vi "eodrecorder.vi"() -> ()   [LabVIEW 2014]
uses:
  eodrecorderstates.ctl
  Control 1.ctl
  <vilib>/Utility/error.llb/DialogType.ctl
  <vilib>/_DAQmxBase/Internals/DAQmxBase Create Channel (AI-Voltage-Basic).vi
  <vilib>/_DAQmxBase/Internals/DAQmxBase Timing (Sample Clock).vi
  <vilib>/_DAQmxBase/Internals/DAQmxBase Read (Analog 2D DBL NChan NSamp).vi
panel:
  out "String 2":string
  out "String":string
  out "Tab Control":enum32{"Live Data", "Edit Data", "View Data"}(tab)
  out "WaveformData":T1
  out "# Pretrigger Samples\nAcquired":i32
  out "Pre-Trigger Error Indicator":bool caption="Error Indicator\n(Indicates if trigger occurs before\npre-trigger samples were acquired)"
  in  "Channel Index":i32
  in  "Pretrigger Samples":i32
  in  "Threshold":sgl
  out "Waveform Graph":dbl[][](graph) caption="Measurement"
  in  "SampleRate":dbl=10000.0
  in  "LiveDataMode":bool
  in  "NumSamptoGrab":i32
  in  "Capture":bool
  in  "Stop":bool
  in  "Open Data":bool
  # "Off"
  # "On"
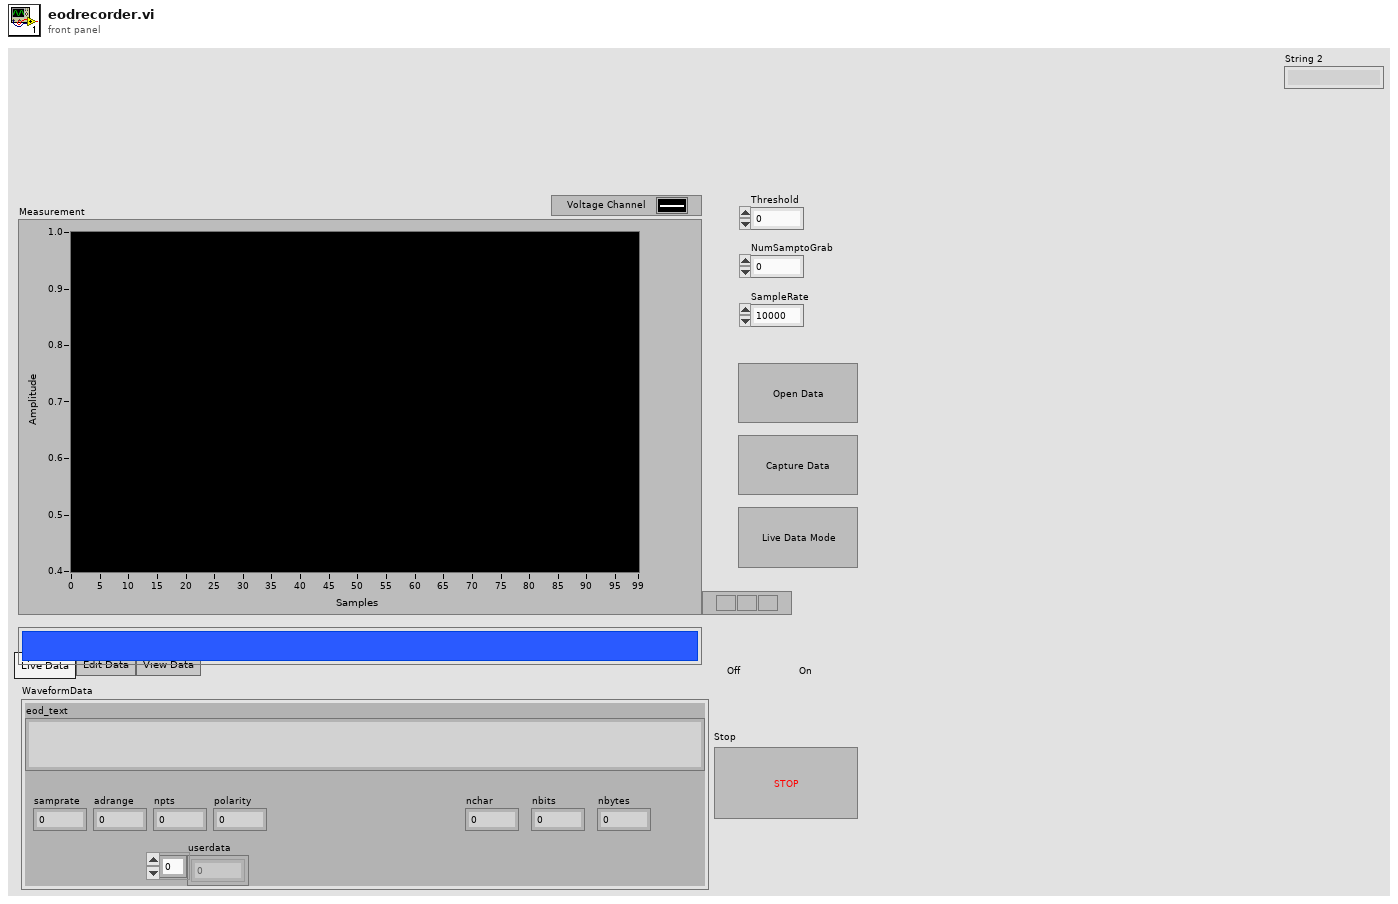
[diagram p1: front panel]
types:
  T1 = cluster{"eod_text":string, "nchar":i32, "nbits":i32, "nbytes":i32, "polarity":i32, "samprate":i32, "adrange":dbl, "userdata":dbl[], "npts":i32, "Wave":dbl[]}
  T2 = cluster{"data":dbl[][], "task ":refnum<k21>, "error ":errorcluster, "Channel":tag, "Min":dbl, "Max":dbl, "Srate":dbl, "WaveformData":cluster{"eod_text":string, "nchar":i32, "nbits":i32, "nbytes":i32, "polarity":i32, "samprate":i32, "adrange":dbl, "userdata":dbl[], "npts":i32, "Wave":dbl[]}}
  T3 = typedef "eodrecorderstates.ctl" = enum16{"stop", "initialize", "live data", "capture data", "analyze data", "open data", "display opened data", "write to file"}
  T4 = typedef "Control 1.ctl" = enum32{"Live Data", "Edit Data", "View Data"}
  T5 = enum16{"Rising Edge", "Falling Edge", "Above Level", "Below Level", "When Inside Window", "When Outside Window"}
  T6 = enum16{"open", "replace", "create", "open or create", "replace or create", "replace or create with confirmation"}
  T7 = typedef "DialogType.ctl" = u16
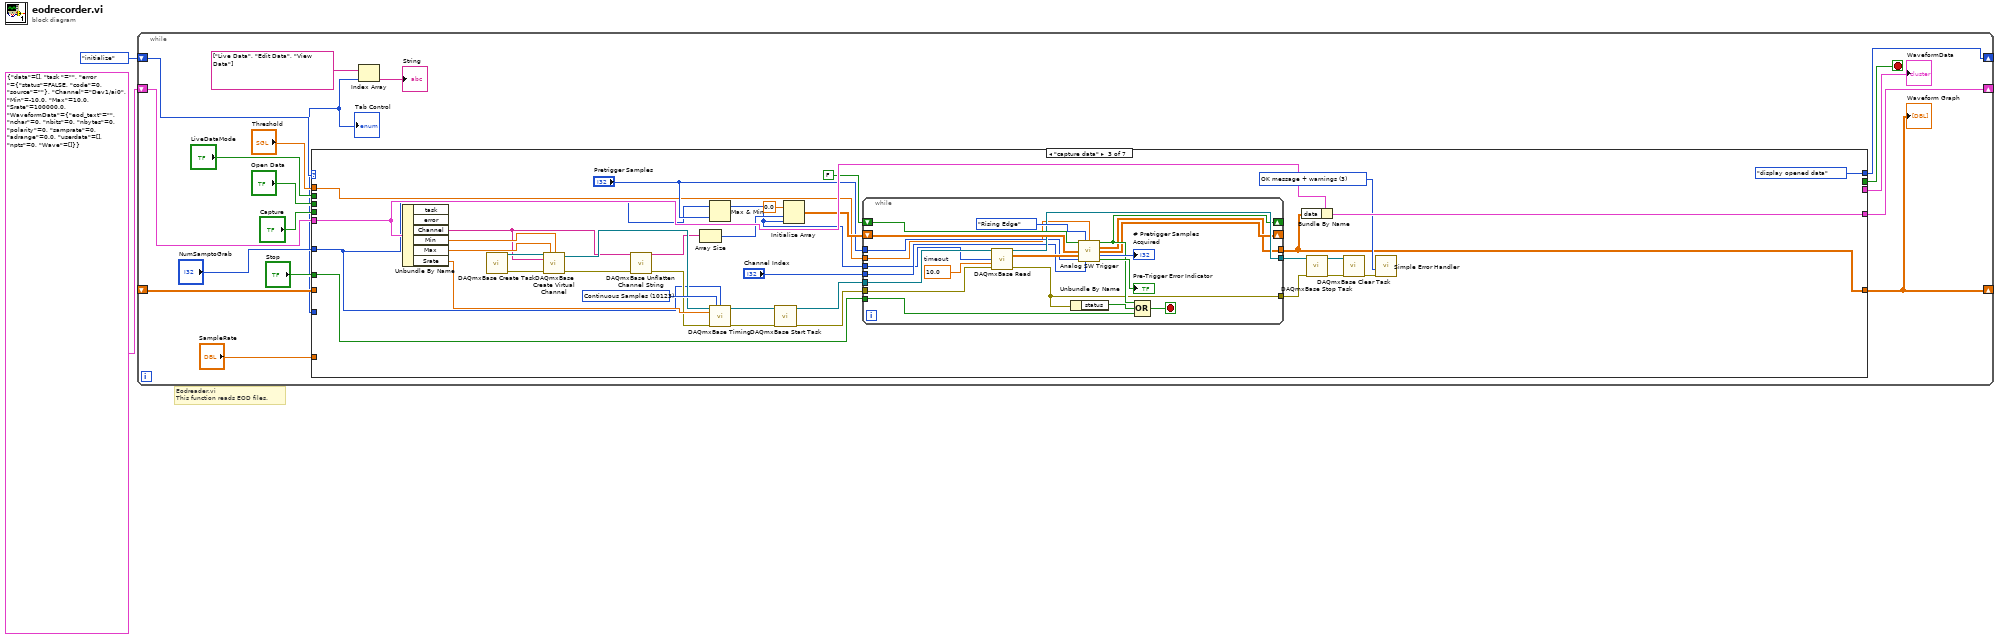
[diagram p0: block diagram]
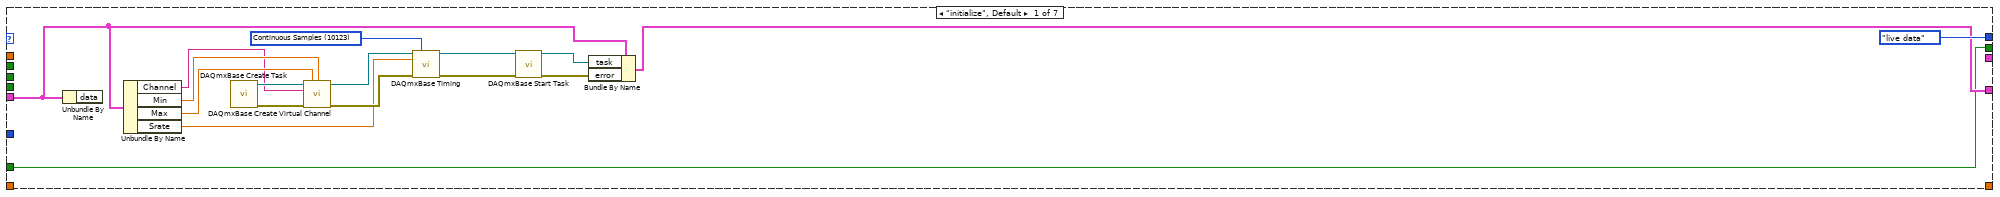
[diagram p2: hidden frame]
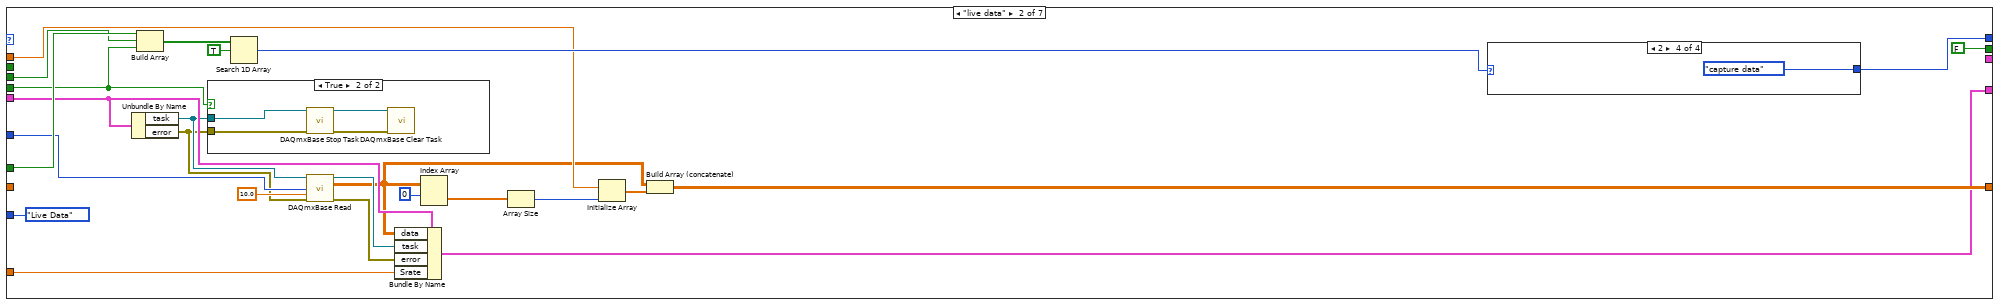
[diagram p3: hidden frame]
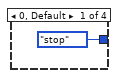
[diagram p5: hidden frame]
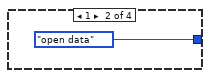
[diagram p6: hidden frame]
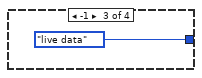
[diagram p7: hidden frame]
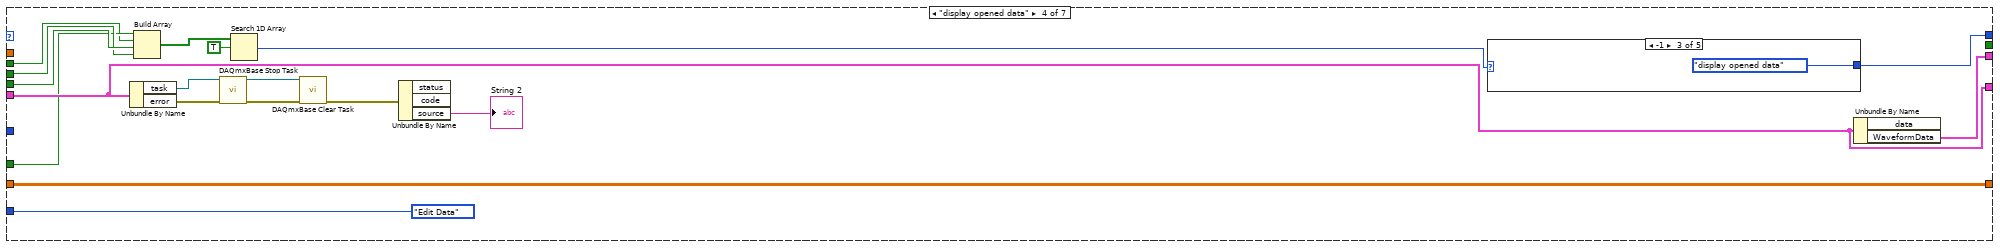
[diagram p8: hidden frame]
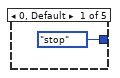
[diagram p9: hidden frame]
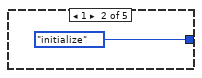
[diagram p10: hidden frame]
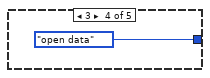
[diagram p11: hidden frame]
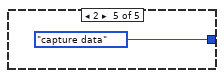
[diagram p12: hidden frame]
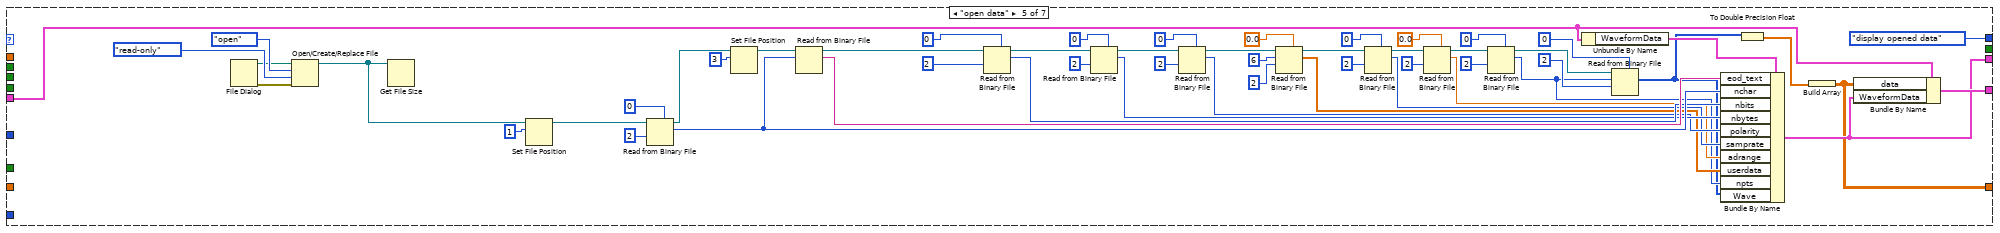
[diagram p13: hidden frame]
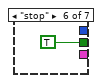
[diagram p14: hidden frame]
diagram:
  # "Eodreader.vi\nThis function reads EOD files."
  n1 = while {
    shift-right: [w19] -> _
    shift-left: eodrecorderstates."initialize" ("Enum") -> [w8]
    shift-right: [w17] -> _
    shift-left: T2 {"data"=[], "task "="", "error "={"status"=FALSE, "code"=0, "source"=""}, "Channel"="Dev1/ai0", "Min"=-10.0, "Max"=10.0, "Srate"=100000.0, "WaveformData"={"eod_text"="", "nchar"=0, "nbits"=0, "nbytes"=0, "polarity"=0, "samprate"=0, "adrange"=0.0, "userdata"=[], "npts"=0, "Wave"=[]}} -> [w14]
    shift-right: [w7] -> _
    shift-left: _ -> [w6]
    stop <- w20 stop-if-true
    n2 = case shown="\"capture data\"" w8 {
      tunnel: [w34 FALSE _ _ _ TRUE _] -> w20
      tunnel: [eodrecorderstates."live data" ("Enum") w61 eodrecorderstates."display opened data" ("Enum") w142 eodrecorderstates."display opened data" ("Enum") _ _] -> w19
      tunnel: "Stop" -> [w34 w60 w74 w136 _ _ _]
      tunnel: w14 -> [w35 w56 w103 w143 w151 _ _]
      tunnel: [w36 w39 w102 w143 w155 _ _] -> w17
      tunnel: [_ _ _ w144 w152 _ _] -> w16
      tunnel: "NumSamptoGrab" -> [_ w52 w71 _ _ _ _]
      tunnel: "SampleRate" -> [_ w50 _ _ _ _ _]
      tunnel: "Open Data" -> [_ w51 _ w138 _ _ _]
      tunnel: "Capture" -> [_ w47 _ w139 _ _ _]
      tunnel: "LiveDataMode" -> [_ _ _ w135 _ _ _]
      tunnel: [_ w48 w72 w128 w150 _ _] -> w7
      tunnel: "Threshold" -> [_ w49 w73 _ _ _ _]
      tunnel: w6 -> [_ _ _ w128 _ _ _]
      tunnel: [_ Control_1."Live Data" ("Tab Control") _ Control_1."Edit Data" ("Tab Control") _ _ _] -> w3
      frame "initialize", Default {
        w29 = 10123 items=["Finite Samples"=10178, "Continuous Samples"=10123] ("sample mode")
        n3 = Unbundle By Name(w35) -> ()  [unwired: 1 out]
        n4 = Unbundle By Name(w35) -> ("Channel"=w21:tag, "Min"=w26:dbl, "Max"=w25:dbl, "Srate"=w24:dbl)
        n5 = call <vilib>:"DAQmxBase Create Task.vi"() -> ("task out"=w32:refnum<k21>, "error out"=w33:errorcluster)  [unwired: 5 in, 9 out]
        n6 = call-poly <vilib>:"DAQmxBase Create Virtual Channel.vi"("task in"=w32, "maximum value"=w25, "minimum value"=w26, "physical channels"=w21, "error in"=w33) -> ("task out"=w30:refnum<k21>, "error out"=w31:errorcluster)  [unwired: 4 in, 5 out]
        n7 = call-poly <vilib>:"DAQmxBase Timing.vi"("task/channels in"=w30, "sample mode"=w29, "rate"=w24, "error in"=w31) -> ("task out"=w23:refnum<k21>, "error out"=w22:errorcluster)  [unwired: 3 in, 7 out]
        n8 = call <vilib>:"DAQmxBase Start Task.vi"("task/channels in"=w23, "error in"=w22) -> ("task out"=w28:refnum<k21>, "error out"=w27:errorcluster)  [unwired: 12 out]
        n9 = Bundle By Name(cluster=w35, "task"=w28, "error"=w27) -> (w36:T2)
      }
      frame "live data" {
        n10 = Unbundle By Name(w56) -> ("task"=w46:refnum<k21>, "error"=w45:errorcluster)
        n11 = Build Array(w60, w51, w47) -> (w59:bool[])
        n12 = case shown="True" w47 {
          tunnel: w46 -> [_ w66]
          tunnel: w45 -> [_ w65]
          frame False {
          }
          frame True {
            n13 = call <vilib>:"DAQmxBase Stop Task.vi"("task/channels in"=w66, "error in"=w65) -> ("task out"=w64:refnum<k21>, "error out"=w63:errorcluster)  [unwired: 12 in]
            n14 = call <vilib>:"DAQmxBase Clear Task.vi"("task in"=w64, "error in"=w63) -> ()  [unwired: 13 in, 1 out]
          }
        }
        n15 = Search 1D Array(1D array=w59, element=TRUE) -> (index of element=w57:i32)  [unwired: 1 in]
        n16 = call-poly <vilib>:"DAQmxBase Read.vi"("task/channels in"=w46, "number of samples per channel"=w52, "timeout"=10.0, "error in"=w45) -> ("task out"=w55:refnum<k21>, "data"=w40:dbl[][], "error out"=w54:errorcluster)  [unwired: 9 out]
        n17 = Bundle By Name(cluster=w56, "data"=w40, "task"=w55, "error"=w54, "Srate"=w50) -> (w39:T2)
        n18 = Index Array(array=w40, index (row)=0) -> (element=w42:dbl[])  [unwired: 1 in]
        n19 = Array Size(array=w42) -> (size(s)=w43:i32)
        n20 = Initialize Array(w49, w43) -> (w41:sgl[])
        n21 = Build Array (concatenate)(w40, w41) -> (w48:dbl[][])
        n22 = case shown="2" w57 {
          tunnel: [eodrecorderstates."stop" ("Enum") eodrecorderstates."open data" ("Enum") eodrecorderstates."live data" ("Enum") eodrecorderstates."capture data" ("Enum")] -> w61
          frame 0, Default {
          }
          frame 1 {
          }
          frame -1 {
          }
          frame 2 {
          }
        }
      }
      frame "capture data" {
        w79 = T7 3 items=["no dialog", "OK message", "continue or stop message", "OK message + warnings", "continue/stop + warnings"] ("type of dialog (OK msg:1)")
        w104 = 10123 items=["Finite Samples"=10178, "Continuous Samples"=10123] ("sample mode")
        n23 = Unbundle By Name(w103) -> ("Channel"=w93:tag, "Min"=w99:dbl, "Max"=w98:dbl, "Srate"=w97:dbl)  [unwired: 2 out]
        n24 = call <vilib>:"DAQmxBase Create Task.vi"() -> ("task out"=w101:refnum<k21>, "error out"=w100:errorcluster)  [unwired: 14 in]
        n25 = call-poly <vilib>:"DAQmxBase Create Virtual Channel.vi"("task in"=w101, "maximum value"=w98, "minimum value"=w99, "physical channels"=w93, "error in"=w100) -> ("task out"=w96:refnum<k21>, "error out"=w92:errorcluster)  [unwired: 9 in]
        n26 = call "DAQmxBase Unflatten Channel String.vi"("names in"=w93, "error in"=w92) -> ("names out"=w90:string[], "error out"=w91:errorcluster)  [unwired: 12 in]
        n27 = Array Size(array=w90) -> (size(s)=w89:i32)
        n28 = Max & Min(x=w71, y="Pretrigger Samples") -> (max(x,y)=w81:i32)  [unwired: 1 out]
        n29 = call-poly <vilib>:"DAQmxBase Timing.vi"("task/channels in"=w96, "sample mode"=w104, "samples per channel"=w71, "rate"=w97, "error in"=w91) -> ("task out"=w95:refnum<k21>, "error out"=w94:errorcluster)  [unwired: 2 in, 7 out]
        n30 = call <vilib>:"DAQmxBase Start Task.vi"("task/channels in"=w95, "error in"=w94) -> ("task out"=w86:refnum<k21>, "error out"=w87:errorcluster)  [unwired: 12 out]
        n31 = Initialize Array(0.0, w89, w81) -> (w85:dbl[][])
        n32 = while {
          tunnel: [w117] -> w76
          shift-right: [w116] -> _
          shift-left: FALSE ("Trigger Out") -> [w125]
          shift-right: [w110] -> _
          shift-left: w85 -> [w119]
          tunnel: w87 -> [w115]
          tunnel: w86 -> [w114]
          tunnel: "Pretrigger Samples" -> [w113]
          tunnel: "Channel Index" -> [w112]
          tunnel: w81 -> [w111]
          tunnel: [w109] -> w72
          tunnel: [w108] -> w75
          tunnel: w74 -> [w107]
          tunnel: w73 -> [w106]
          stop <- w123 stop-if-true
          w126 = 10.0  # timeout
          n33 = call-poly <vilib>:"DAQmxBase Read.vi"("task/channels in"=w114, "number of samples per channel"=w111, "timeout"=w126, "error in"=w115) -> ("task out"=w117:refnum<k21>, "data"=w120:dbl[][], "error out"=w108:errorcluster)  [unwired: 9 in]
          n34 = Unbundle By Name(w108) -> ("status"=w124:bool)
          n35 = call "Analog SW Trigger.vi"("Triggered?"=w125, "Condition"=T5."Rising Edge", "Level"=w106, "Initialized Data Array"=w119, "Input Raw Data"=w120, "Pretrigger Samples"=w113, "Index of Condition Channel"=w112) -> ("Trigger Out"=w116:bool, "Output Data (Scaled)"=w109:dbl[][], "Raw Data Out"=w110:dbl[][], "# Pretrigger Samples"=→"# Pretrigger Samples\nAcquired":i32, "Pre-Trigger Error"=→"Pre-Trigger Error Indicator":bool)  [unwired: 4 in]
          n36 = Compound Arithmetic op=OR(w116, w124, w107) -> (w123:bool)
        }
        n37 = Bundle By Name(cluster=w103, "data"=w72) -> (w102:T2)
        n38 = call <vilib>:"DAQmxBase Stop Task.vi"("task/channels in"=w76, "error in"=w75) -> ("task out"=w78:refnum<k21>, "error out"=w77:errorcluster)  [unwired: 12 in]
        n39 = call <vilib>:"DAQmxBase Clear Task.vi"("task in"=w78, "error in"=w77) -> ("error out"=w80:errorcluster)  [unwired: 13 in]
        n40 = call <vilib>:"Simple Error Handler.vi"("type of dialog (OK msg:1)"=w79, "error in (no error)"=w80) -> ()  [unwired: 3 in, 5 out]
      }
      frame "display opened data" {
        n41 = Unbundle By Name(w143) -> ("task"=w130:refnum<k21>, "error"=w129:errorcluster)
        n42 = Build Array(w136, w135, w139, w138) -> (w141:bool[])
        n43 = call <vilib>:"DAQmxBase Stop Task.vi"("task/channels in"=w130, "error in"=w129) -> ("task out"=w131:refnum<k21>, "error out"=w132:errorcluster)  [unwired: 12 in]
        n44 = Search 1D Array(1D array=w141, element=TRUE) -> (index of element=w137:i32)  [unwired: 1 in]
        n45 = call <vilib>:"DAQmxBase Clear Task.vi"("task in"=w131, "error in"=w132) -> ("error out"=w133:errorcluster)  [unwired: 13 in]
        n46 = Unbundle By Name(w133) -> ("source"=→"String 2":string)  [unwired: 2 out]
        n47 = case shown="-1" w137 {
          tunnel: [eodrecorderstates."stop" ("Enum") eodrecorderstates."initialize" ("Enum") eodrecorderstates."display opened data" ("Enum") eodrecorderstates."open data" ("Enum") eodrecorderstates."capture data" ("Enum")] -> w142
          frame 0, Default {
          }
          frame 1 {
          }
          frame -1 {
          }
          frame 3 {
          }
          frame 2 {
          }
        }
        n48 = Unbundle By Name(w143) -> ("WaveformData"=w144:T1)  [unwired: 1 out]
      }
      frame "open data" {
        n49 = File Dialog() -> (0:w199:errorcluster, 3:w200:path)  [unwired: 7 in, 2 out]
        n50 = Open/Create/Replace File(file path (use dialog)=w200, error in=w199, operation (0:open)=T6."open", access (0:read/write)=enum16{"read/write", "read-only", "write-only"}."read-only") -> (refnum out=w198:refnum<file>)  [unwired: 2 in, 2 out]
        n51 = Get File Size(file=w198) -> ()  [unwired: 1 in, 3 out]
        n52 = Set File Position(offset (in bytes) (0)=1, refnum=w198) -> (refnum out=w196:refnum<file>)  [unwired: 2 in, 1 out]
        n53 = Read from Binary File(5:u8 0, 9:2, 11:w196) -> (2:w165:u8, 3:w194:refnum<file>)  [unwired: 3 in, 2 out]
        n54 = Set File Position(offset (in bytes) (0)=3, refnum=w194) -> (refnum out=w192:refnum<file>)  [unwired: 2 in, 1 out]
        n55 = Read from Binary File(10:w165, 11:w192) -> (2:w164:string, 3:w191:refnum<file>)  [unwired: 4 in, 2 out]
        n56 = Read from Binary File(5:i8 0, 9:2, 11:w191) -> (2:w163:i8, 3:w167:refnum<file>)  [unwired: 3 in, 2 out]
        n57 = Read from Binary File(5:i8 0, 9:2, 11:w167) -> (2:w162:i8, 3:w168:refnum<file>)  [unwired: 3 in, 2 out]
        n58 = Read from Binary File(5:i8 0, 9:2, 11:w168) -> (2:w161:i8, 3:w166:refnum<file>)  [unwired: 3 in, 2 out]
        n59 = Read from Binary File(5:sgl 0.0, 9:2, 10:6, 11:w166) -> (2:w160:sgl[], 3:w188:refnum<file>)  [unwired: 2 in, 2 out]
        n60 = Read from Binary File(5:u32 0, 9:2, 11:w188) -> (2:w159:u32, 3:w180:refnum<file>)  [unwired: 3 in, 2 out]
        n61 = Read from Binary File(5:sgl 0.0, 9:2, 11:w180) -> (2:w158:sgl, 3:w174:refnum<file>)  [unwired: 3 in, 2 out]
        n62 = Read from Binary File(5:u32 0, 9:2, 11:w174) -> (2:w157:u32, 3:w175:refnum<file>)  [unwired: 3 in, 2 out]
        n63 = Unbundle By Name(w151) -> ("WaveformData"=w156:T1)
        n64 = Read from Binary File(5:0, 9:2, 10:w157, 11:w175) -> (2:w154:i32[])  [unwired: 2 in, 3 out]
        n65 = Bundle By Name(cluster=w156, "eod_text"=w164, "nchar"=w165, "nbits"=w163, "nbytes"=w162, "polarity"=w161, "samprate"=w159, "adrange"=w158, "userdata"=w160, "npts"=w157, "Wave"=w154) -> (w152:T1)
        n66 = To Double Precision Float(number=w154) -> (double precision float=w153:dbl[])
        n67 = Build Array(w153) -> (w150:dbl[][])
        n68 = Bundle By Name(cluster=w151, "data"=w150, "WaveformData"=w152) -> (w155:T2)
      }
      frame "stop" {
      }
      frame "analyze data" {
      }
    }
    "WaveformData" <- w16
    "Waveform Graph" <- w7
    "Tab Control" <- w3
    n69 = Index Array(array=string[] ["Live Data", "Edit Data", "View Data"], index=w3) -> (element=→"String":string)
  }
